vi "Acquisition Increment.vi"(8 "error in (no error)":errorcluster, 11 "Top Level in":refnum<class "Top Level.lvclass">) -> (0 "error out":errorcluster, 3 "Top Level out":refnum<class "Top Level.lvclass">)   [LabVIEW 2021, in "Top Level.lvlib" / "Top Level.lvclass"]
uses:
  Top Level.lvclass
  Top Level.lvclass/Top Level.ctl
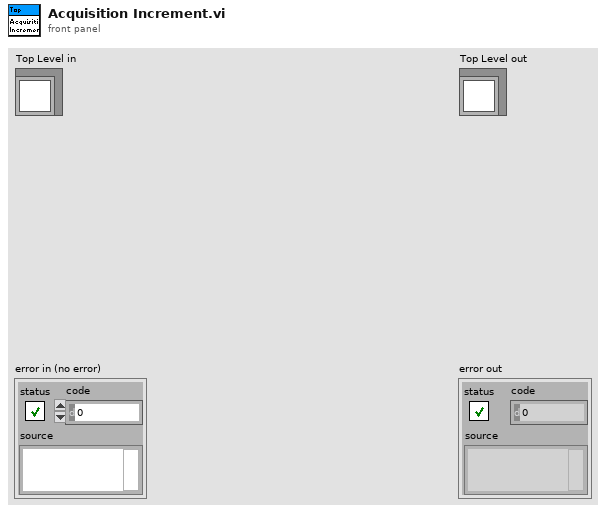
[diagram p1: front panel]
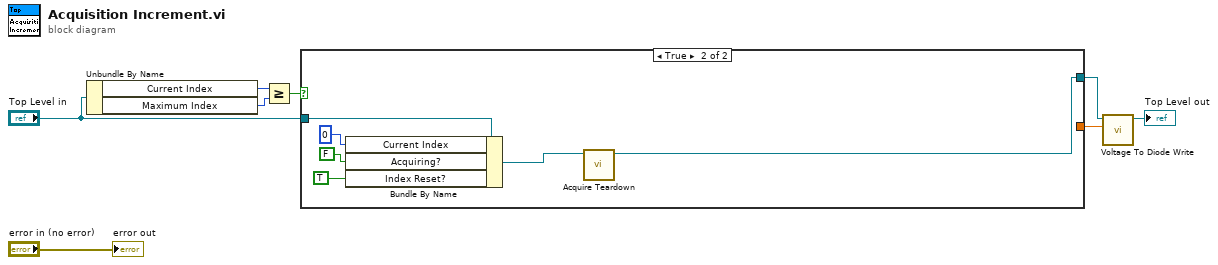
[diagram p0: block diagram]
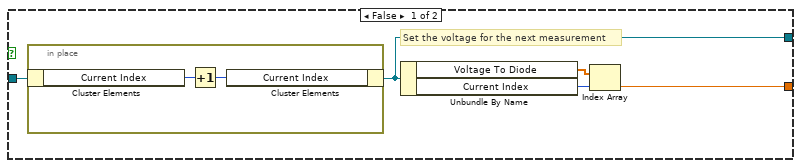
[diagram p2: hidden frame]
diagram:
  n1 = Unbundle By Name("Top Level in") -> ("Current Index"=w5:i32, "Maximum Index"=w6:i32)
  n2 = Greater Or Equal?(x=w5, y=w6) -> (x >= y?=w4:bool)
  n3 = case shown="True" w4 {
    tunnel: "Top Level in" -> [w13 w21]
    tunnel: [w10 w17] -> w3
    tunnel: [w9 _] -> w1
    frame False {
      # "Set the voltage for the next measurement"
      n4 = in-place {
        n5 = in-place-cluster #1(w13) -> ("Current Index"=w14:i32)
        n6 = Increment(x=w14) -> (x+1=w15:i32)
        n7 = in-place-cluster #1("Current Index"=w15) -> (w10:refnum<class "Top Level.lvclass">)
      }
      n8 = Unbundle By Name(w10) -> ("Voltage To Diode"=w12:dbl[], "Current Index"=w11:i32)
      n9 = Index Array(array=w12, index=w11) -> (element=w9:dbl)
    }
    frame True {
      n10 = Bundle By Name(cluster=w21, "Current Index"=0 ("Acquisition.Current Index"), "Acquiring?"=FALSE, "Index Reset?"=TRUE) -> (w18:refnum<class "Top Level.lvclass">)
      n11 = call "Acquire Teardown.vi"("Top Level in"=w18) -> ("Top Level out"=w17:refnum<class "Top Level.lvclass">)  [unwired: 9 in, 1 out]
    }
  }
  n12 = call "Voltage To Diode Write.vi"("Voltage"=w1, "Top Level in"=w3) -> ("Top Level out"=→"Top Level out":refnum<class "Top Level.lvclass">)  [unwired: 8 in, 1 out]
  "error out" <- "error in (no error)"
